vi "LED Test.vi"() -> ()   [LabVIEW 2020]
uses:
  <vilib>/MakerHub/LINX/Private/Device/Type Defs/TCP Config.ctl
  <vilib>/MakerHub/LINX/Public/Peripherals/Digital/Digital Write 1 Chan.vi
  <vilib>/MakerHub/LINX/Public/Peripherals/Digital/Digital Write N Chans.vi
  <vilib>/MakerHub/LINX/Private/Local IO/LinxDigitalWrite.vi
  <vilib>/MakerHub/LINX/Public/Utilities/Check Channel.vi
  <vilib>/MakerHub/LINX/Public/Utilities/Open Serial.vi
  <vilib>/MakerHub/LINX/Public/Utilities/Open TCP.vi
  <vilib>/MakerHub/LINX/Private/Utilties/Generate Error.vi
  <vilib>/MakerHub/LINX/LMH-LINX.lvlib
  <vilib>/MakerHub/LINX/Private/Device/Device.lvlib
panel:
  in  "TCP Configuration":T1={"IP Address"="0.0.0.0", "Port"=44300}
  in  "Use TCP":bool
  in  "Stop Button":bool
  in  "LED":bool
  out "Loop Rate (Hz)":u32
  in  "Serial Port":refnum<visa-resource-name>
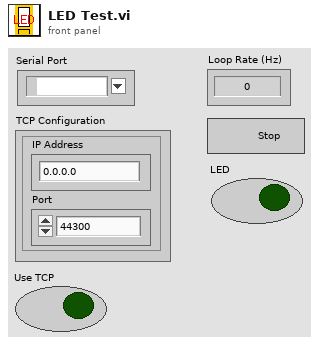
[diagram p1: front panel]
types:
  T1 = typedef "LMH-LINX.lvlib/Device.lvlib/TCP Config.ctl" = cluster{"IP Address":string, "Port":u16}
  T2 = typedef "LMH-LINX.lvlib/LINX Ref.ctl" = cluster{"IO":T3, "Interface":T4, "LINX Device Config":T5}
  T3 = typedef "LMH-LINX.lvlib/Platform.ctl" = enum16{"Remote", "Local"}
  T4 = typedef "LMH-LINX.lvlib/Interface.ctl" = enum16{"Serial", "TCP"}
  T5 = typedef "LMH-LINX.lvlib/Device.lvlib/LINX Device Config.ctl" = cluster{"Interface":T4, "COM Port":refnum<visa-resource-name>, "TCP Configuration":T1, "Device Family":u8, "Device ID":u8, "Device Name":string, "TCP Ref":refnum<k5>, "Channels":T6}
  T6 = typedef "LMH-LINX.lvlib/Channels.ctl" = cluster{"DI":u8[], "DO":u8[], "AI":u8[], "AO":u8[], "PWM":u8[], "QE":u8[], "UART":u8[], "I2C 2":u8[], "SPI":u8[], "CAN":u8[], "Servo":u8[], "AI Ref (V)":dbl, "AI Resolution (Bits)":u8, "AO Ref (V)":dbl, "AO Resolution (Bits)":u8}
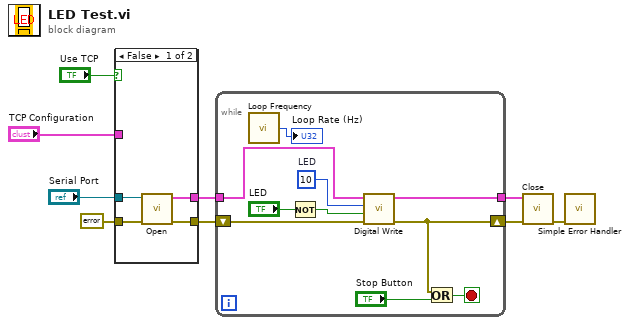
[diagram p0: block diagram]
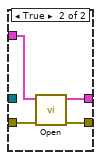
[diagram p2: hidden frame]
diagram:
  n1 = case shown="False" "Use TCP" {
    tunnel: [w11 w17] -> w9
    tunnel: [w12 w16] -> w8
    tunnel: errorcluster {"status"=FALSE, "code"=0, "source"=""} ("Error In") -> [w13 w15]
    tunnel: "Serial Port" -> [w10 _]
    tunnel: "TCP Configuration" -> [_ w14]
    frame False {
      n2 = call-poly <vilib>:"Open.vi"("Error In"=w13, "Serial Port"=w10) -> ("Error Out"=w12:errorcluster, "LINX Resource"=w11:T2)  [unwired: 7 in, 1 out]
    }
    frame True {
      n3 = call-poly <vilib>:"Open.vi"("Error In"=w15, "TCP Configuration"=w14) -> ("Error Out"=w16:errorcluster, "LINX Resource"=w17:T2)  [unwired: 7 in, 1 out]
    }
  }
  n4 = while {
    tunnel: w9 -> [w25]
    tunnel: [w24] -> w7
    shift-right: [w22] -> w6
    shift-left: w8 -> [w23]
    stop <- w27 stop-if-true
    w20 = u8 10  # LED
    n5 = call <vilib>:"Loop Frequency.vi"() -> ("Loop Rate (Hz)"=→"Loop Rate (Hz)":u32)
    n6 = Not(x="LED") -> (.not. x?=w19:bool)
    n7 = call-poly <vilib>:"Digital Write.vi"("Error In"=w23, "Output Value"=w19, "DO Channel"=w20, "LINX Resource"=w25) -> ("Error Out"=w22:errorcluster, "LINX Resource"=w24:T2)  [unwired: 6 in]
    n8 = Or(x=w22, y="Stop Button") -> (x .or. y?=w27:bool)
  }
  n9 = call <vilib>:"Close.vi"("Error In"=w6, "LINX Resource"=w7) -> ("Error Out"=w5:errorcluster)  [unwired: 9 in]
  n10 = call <vilib>:"Simple Error Handler.vi"("error in (no error)"=w5) -> ()  [unwired: 4 in, 5 out]
